vi "UI Subpanel.vi"() -> ()   [LabVIEW 2021, in "CIF Template UI.lvlib"]
uses:
  CIF Template UI.lvlib
  Common/Typedef/Configuration.ctl
  CIF-LVCore/src/CIFCore/Common/Typedef/Common Plugin Configuration.ctl
  CIF-LVCore/src/CIFUI/Typedef/Class Data for SubPanel.ctl
  <vilib>/gRPC/LabVIEW gRPC Library/Shared/grpcId.ctl
  CIF-LVCore/src/CIFUI/Typedef/Core UI References.ctl
  CIF-LVCore/src/CIFUI/Typedef/Channel Connection.ctl
  CIF-LVCore/src/CIFUI/Typedef/New Plugin.ctl
  CIF-LVCore/src/CIFUI/Typedef/Run Listen Button.ctl
  CIF-LVCore/src/CIFUI/Typedef/CIF_Manager_UI_Tab.ctl
  CIF-LVCore/src/CIFUI/Typedef/SubPanel Events.ctl
  CIF-LVCore/src/CIFUI/Typedef/New Connection Event Data.ctl
  CIF-LVCore/src/CIFUI/Typedef/New Connection Plugin Event Data.ctl
  CIF-LVCore/src/CIFUI/CIF_UI.lvclass
  CIF-LVCore/src/CIFUI/CIF_UI.lvclass/CIF_UI.ctl
  CIF-LVCore/src/CIFUI/Utilities/Get Human Readable Error.vi
  Grpc/Template_wrapper/TemplateWrapper.lvlib
  <vilib>/addons/_JKI.lib/Serialization/JSON/JKI JSON Serialization.lvlib
  CIF-LVCore/src/CIFCore/Grpc/CIFCoreWrapper/CIFCoreWrapper.lvlib
  CIF-LVCore/src/CIFCore/Common/CIFCoreCommon.lvlib
  Common/TemplateCommon.lvlib
  <vilib>/gRPC/LabVIEW gRPC Library/grpc-lvsupport-release.lvlib
panel:
  in  "Class Data for SubPanel":T1
  in  "Update Config":bool
  in  "Configuration":T5={"Common"={"Period (s)"=0.001, "Offset (us)"=0, "ClockID"=0, "Priority"=100, "Processor"=-2}, "Step"=100} {"Common"."Period (s)" format="%#_13g"}
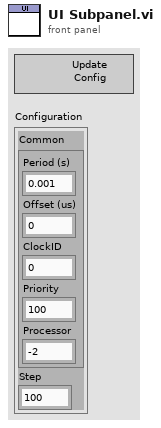
[diagram p1: front panel]
types:
  T1 = typedef "CIF_UI.lvclass/Class Data for SubPanel.ctl" = cluster{"IP Address":string, "Manager gRPC ID":T2, "Server Certificate File (.crt)":path, "Connected":bool, "Manager Connection":bool, "Core UI References":T3, "Subpanel Events":T4}
  T2 = typedef "grpc-lvsupport-release.lvlib/grpcId.ctl" = u64
  T3 = typedef "CIF_UI.lvclass/Core UI References.ctl" = cluster{"Discovered Plugins":refnum<vi>, "Discovered Plugins Valid":bool, "Loaded Plugins":refnum<vi>, "Loaded Plugins Valid":bool, "Publisher Channels":refnum<vi>, "Publisher Channels Valid":bool, "Subscriber Channels":refnum<vi>, "Subscriber Channels Valid":bool, "Plugin Status":refnum<vi>, "Plugin Status Valid":bool, "Channel Connection":refnum<vi>, "Channel Connection Valid":bool, "New Plugin Load":refnum<vi>, "New Plugin Load Valid":bool, "Errors":refnum<vi>, "Errors Valid":bool, "Plugin to Abort":refnum<vi>, "Plugin to Abort Valid":bool, "Connection":refnum<vi>, "Connection Valid":bool, "Exit":refnum<vi>, "Exit Valid":bool, "Run Listen":refnum<vi>, "Run Listen Valid":bool, "CIF Manager Tab":refnum<vi>, "Manger Tab Valid":bool, "Clear Local Error":refnum<vi>, "Clear Local Error Valid":bool, "Local Error":refnum<vi>, "Local Error Valid":bool, "System Errors":refnum<vi>, "System Errors Valid":bool, "Plugin Selection":refnum<vi>, "Plugin Selection Valid":bool}
  T4 = typedef "CIF_UI.lvclass/SubPanel Events.ctl" = cluster{"Clear Local Error":refnum<user-event>, "Shutdown":refnum<user-event>, "gRPC Connection":refnum<user-event>, "Plugin Connection":refnum<user-event>}
  T5 = typedef "TemplateCommon.lvlib/Configuration.ctl" = cluster{"Common":T6, "Step":u64}
  T6 = typedef "CIFCoreCommon.lvlib/Common Plugin Configuration.ctl" = cluster{"Period (s)":dbl, "Offset (us)":i32, "ClockID":u8, "Priority":i32, "Processor":i32}
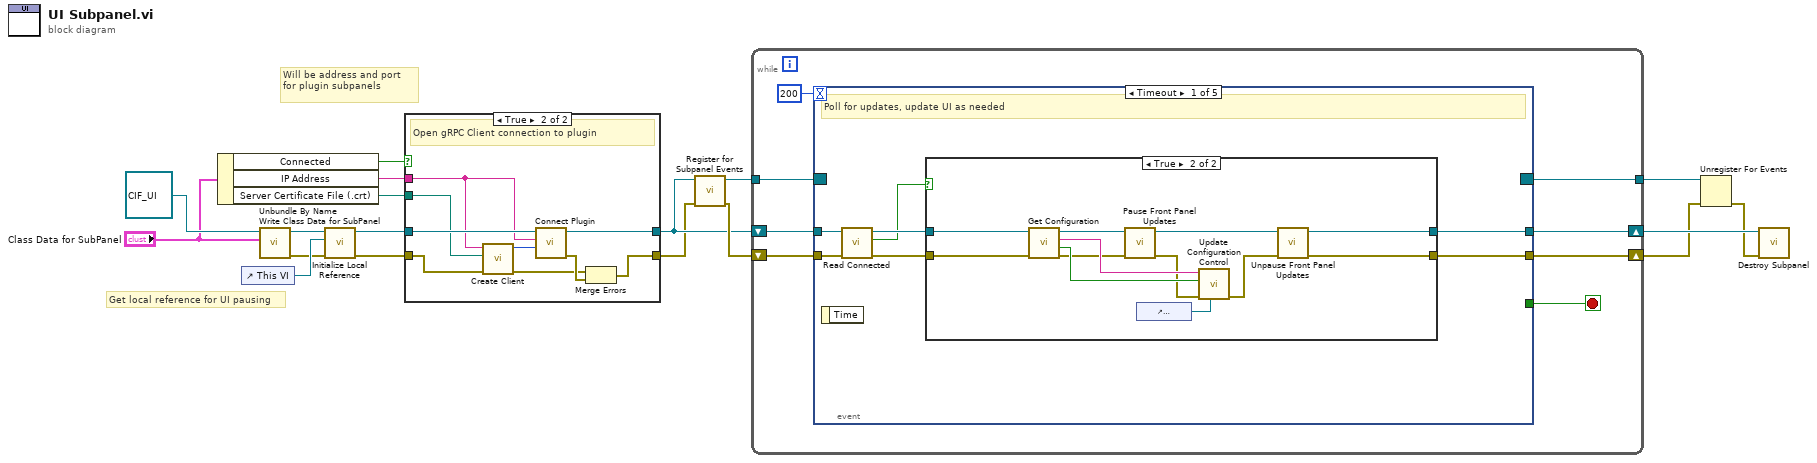
[diagram p0: block diagram]
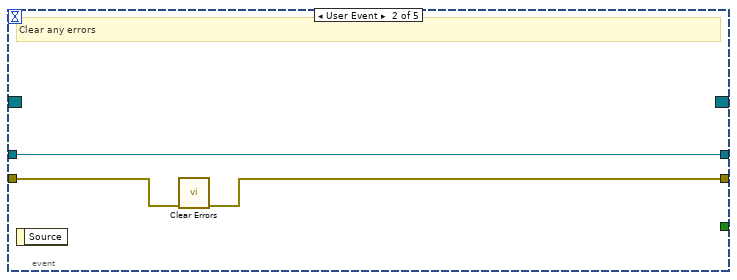
[diagram p4: hidden frame]
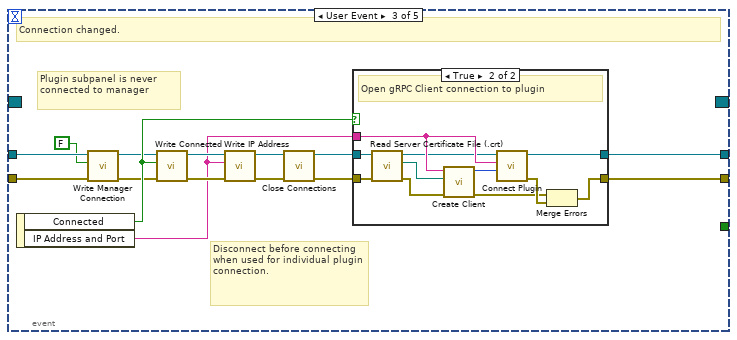
[diagram p5: hidden frame]
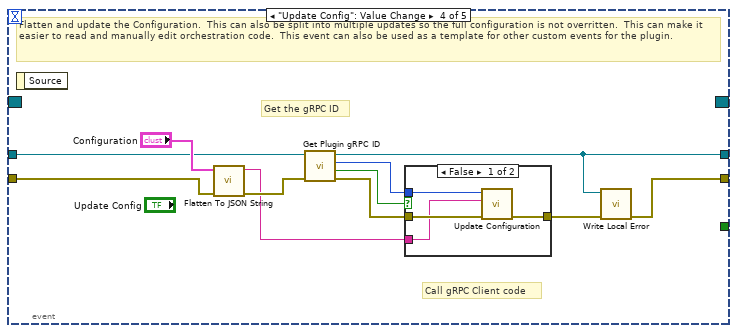
[diagram p7: hidden frame]
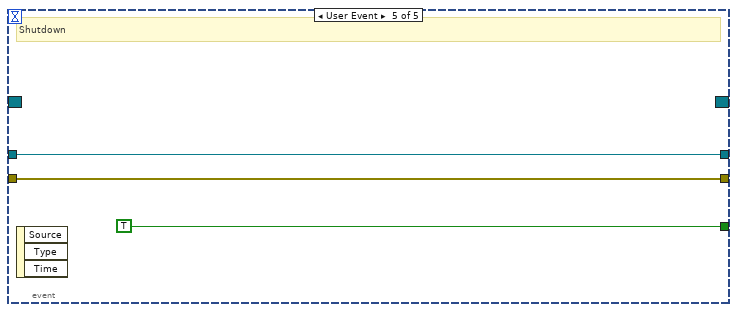
[diagram p9: hidden frame]
diagram:
  # "Will be address and port for plugin subpanels"
  # "Get local reference for UI pausing"
  n1 = Unbundle By Name("Class Data for SubPanel") -> ("Connected"=w3:bool, "IP Address"=w2:string, "Server Certificate File (.crt)"=w1:path)
  n2 = control-ref of="This VI"() -> (w18:refnum<vi>)
  n3 = call "Write Class Data for SubPanel.vi"("Class Data for SubPanel"="Class Data for SubPanel", "CIF_UI in"=refnum<class "CIF_UI.lvclass"> refnum) -> ("error out"=w9:errorcluster, "CIF_UI out"=w11:refnum<class "CIF_UI.lvclass">)  [unwired: 8 in]
  n4 = call "Initialize Local Reference.vi"("error in (no error)"=w9, "This VI"=w18, "CIF_UI in"=w11) -> ("error out"=w7:errorcluster, "CIF_UI out"=w8:refnum<class "CIF_UI.lvclass">)  [unwired: 7 in]
  n5 = case shown="True" w3 {
    tunnel: [w19 w29] -> w5
    tunnel: [w20 w27] -> w6
    tunnel: w8 -> [w20 w26]
    tunnel: w7 -> [w19 w25]
    tunnel: w2 -> [_ w22]
    tunnel: w1 -> [_ w21]
    frame False {
    }
    frame True {
      # "Open gRPC Client connection to plugin"
      n6 = call "Create Client.vi"("error in"=w25, "Server Certificate File (.crt)"=w21, "address"=w22) -> ("error out"=w24:errorcluster, "gRPC ID Out"=w23:T2)  [unwired: 7 in]
      n7 = call "Connect Plugin.vi"("gRPC ID"=w23, "Address"=w22, "CIF_UI in"=w26) -> ("error out"=w28:errorcluster, "CIF_UI out"=w27:refnum<class "CIF_UI.lvclass">)  [unwired: 7 in]
      n8 = Merge Errors(w24, w28) -> (w29:errorcluster)
    }
  }
  n9 = call "Register for Subpanel Events.vi"("error in (no error)"=w5, "CIF_UI in"=w6) -> ("error out"=w16:errorcluster, "Event Registration Refnum"=w17:refnum<event-registration>)  [unwired: 8 in]
  n10 = while {
    tunnel: w17 -> [w36]
    shift-right: [w31] -> w15
    shift-left: w6 -> [w34]
    shift-right: [w32] -> w13
    shift-left: w16 -> [w33]
    tunnel: [w30] -> w14
    stop <- w35 stop-if-true
    n11 = event shown="[0] Timeout" {
      selector: w36 -> [_ _ _ _ _]
      dyn-events: [_ _ _ _ _] -> w30
      timeout: 200 -> [_ _ _ _ _]
      tunnel: [_ _ _ _ TRUE] -> w35
      tunnel: w34 -> [w40 w59 w66 w94 w107]
      tunnel: w33 -> [w41 w61 w65 w99 w106]
      tunnel: [w38 w60 w67 w98 w106] -> w32
      tunnel: [w39 w59 w68 w91 w107] -> w31
      event Timeout {
        # "Poll for updates, update UI as needed"
        n12 = event-data() -> ()  [unwired: 1 in, 1 out]
        n13 = call "Read Connected.vi"("error in (no error)"=w41, "CIF_UI in"=w40) -> ("error out"=w43:errorcluster, "Connected"=w42:bool, "CIF_UI out"=w44:refnum<class "CIF_UI.lvclass">)  [unwired: 7 in]
        n14 = case shown="True" w42 {
          tunnel: w43 -> [w45 w51]
          tunnel: [w45 w58] -> w38
          tunnel: w44 -> [w46 w52]
          tunnel: [w46 w57] -> w39
          frame False {
          }
          frame True {
            n15 = call "Get Configuration.vi"("error in (no error)"=w51, "CIF_Plugin_UI in"=w52) -> ("error out"=w49:errorcluster, "Not Found"=w54:bool, "JSON Configuration"=w55:string, "CIF_Plugin_UI out"=w50:refnum<class "CIF_UI.lvclass">)  [unwired: 6 in]
            n16 = call "Pause Front Panel Updates.vi"("error in (no error)"=w49, "CIF_UI in"=w50) -> ("error out"=w48:errorcluster, "CIF_UI out"=w47:refnum<class "CIF_UI.lvclass">)  [unwired: 8 in]
            n17 = control-ref of="Configuration"() -> (w53:refnum<vi>)
            n18 = call "Update Configuration Control.vi"("Configuration reference"=w53, "error in (no error)"=w48, "Not Valid"=w54, "JSON Configuration"=w55) -> ("error out"=w56:errorcluster)  [unwired: 7 in]
            n19 = call "Unpause Front Panel Updates.vi"("error in (no error)"=w56, "CIF_UI in"=w47) -> ("error out"=w58:errorcluster, "CIF_UI out"=w57:refnum<class "CIF_UI.lvclass">)  [unwired: 8 in]
          }
        }
      }
      event User Event {
        # "Clear any errors"
        n20 = event-data() -> ()  [unwired: 1 in, 1 out]
        n21 = call <vilib>:"Clear Errors.vi"("error in (no error)"=w61) -> ("error out"=w60:errorcluster)  [unwired: 5 in, 1 out]
      }
      event User Event {
        # "Plugin subpanel is never connected to manager"
        # "Disconnect before connecting when used for individual plugin connection."
        # "Connection changed."
        n22 = event-data() -> ("Connected"=w69:bool, "IP Address and Port"=w70:string)  [unwired: 1 in]
        n23 = call "Write Manager Connection.vi"("error in (no error)"=w65, "Manager Connection"=FALSE, "CIF_UI in"=w66) -> ("error out"=w63:errorcluster, "CIF_UI out"=w64:refnum<class "CIF_UI.lvclass">)  [unwired: 7 in]
        n24 = call "Write Connected.vi"("error in (no error)"=w63, "Connected"=w69, "CIF_UI in"=w64) -> ("error out"=w75:errorcluster, "CIF_UI out"=w76:refnum<class "CIF_UI.lvclass">)  [unwired: 7 in]
        n25 = call "Write IP Address.vi"("error in (no error)"=w75, "IP Address"=w70, "CIF_UI in"=w76) -> ("error out"=w73:errorcluster, "CIF_UI out"=w74:refnum<class "CIF_UI.lvclass">)  [unwired: 7 in]
        n26 = call "Close Connections.vi"("error in (no error)"=w73, "CIF_UI in"=w74) -> ("error out"=w71:errorcluster, "CIF_UI out"=w72:refnum<class "CIF_UI.lvclass">)  [unwired: 8 in]
        n27 = case shown="True" w69 {
          tunnel: [w77 w89] -> w67
          tunnel: [w78 w87] -> w68
          tunnel: w72 -> [w78 w83]
          tunnel: w71 -> [w77 w82]
          tunnel: w70 -> [_ w84]
          frame False {
          }
          frame True {
            # "Open gRPC Client connection to plugin"
            n28 = call "Read Server Certificate File (.crt).vi"("error in (no error)"=w82, "CIF_UI in"=w83) -> ("error out"=w80:errorcluster, "Server Certificate File (.crt)"=w79:path, "CIF_UI out"=w81:refnum<class "CIF_UI.lvclass">)  [unwired: 7 in]
            n29 = call "Create Client.vi"("error in"=w80, "Server Certificate File (.crt)"=w79, "address"=w84) -> ("error out"=w86:errorcluster, "gRPC ID Out"=w85:T2)  [unwired: 7 in]
            n30 = call "Connect Plugin.vi"("gRPC ID"=w85, "Address"=w84, "CIF_UI in"=w81) -> ("error out"=w88:errorcluster, "CIF_UI out"=w87:refnum<class "CIF_UI.lvclass">)  [unwired: 7 in]
            n31 = Merge Errors(w86, w88) -> (w89:errorcluster)
          }
        }
      }
      event "Update Config": Value Change {
        # "Call gRPC Client code"
        # "Get the gRPC ID"
        # "Flatten and update the Configuration.  This can also be split into multiple updates so the full configuration is not overritten.  This can make it easier to read and manually edit orchestration code.  This event can also be used as a template for other custom events for the plugin."
        n32 = event-data() -> ()  [unwired: 1 in, 1 out]
        n33 = call <vilib>:"Flatten To JSON String.vi"("error in (no error)"=w99, "Variant"="Configuration") -> ("error out"=w93:errorcluster, "JSON String"=w92:string)  [unwired: 8 in]
        n34 = call "Get Plugin gRPC ID.vi"("error in (no error)"=w93, "CIF_UI in"=w94) -> ("error out"=w95:errorcluster, "Not Found"=w96:bool, "gRPC ID"=w97:T2, "CIF_UI out"=w91:refnum<class "CIF_UI.lvclass">)  [unwired: 5 in, 1 out]
        n35 = case shown="False" w96 {
          tunnel: w97 -> [w104 _]
          tunnel: w95 -> [w103 w105]
          tunnel: [w102 w105] -> w90
          tunnel: w92 -> [w101 _]
          frame False {
            n36 = call "Update Configuration.vi"("error in"=w103, "JSON Configuration"=w101, "gRPC ID"=w104) -> ("error out"=w102:errorcluster)  [unwired: 7 in, 1 out]
          }
          frame True {
          }
        }
        n37 = call "Write Local Error.vi"("error in (no error)"=w90, "CIF_UI in"=w91) -> ("error out"=w98:errorcluster)  [unwired: 9 in]
      }
      event User Event {
        # "Shutdown"
        n38 = event-data() -> ()  [unwired: 1 in, 3 out]
      }
    }
  }
  n39 = Unregister For Events(event registration refnum=w14, error in=w13) -> (error out=w12:errorcluster)
  n40 = call "Destroy Subpanel.vi"("error in (no error)"=w12, "CIF_UI in"=w15) -> ()  [unwired: 8 in, 2 out]
